vi "EJERCICIO 3.vi"() -> ()   [LabVIEW 2014]
uses:
  Tabcontrolcajero.ctl
  Control 1.ctl
panel:
  out "Tab Control":T1
  out "String 2":string
  out "String":string
  out "Boolean 3":bool
  in  "CARD":bool
  in  "picture":picture
  in  "picture 3":picture
  in  "picture 2":picture
  out "String 3":string
  out "Horizontal Progress Bar":dbl(slide) scale=0.0..100.0
  out "decimal integer string":string
  out "String 4":string
  in  "Contraseña":string
  in  "Aceptar":bool
  out "s? t:f":string
  out "s? t:f 3":string
  out "s? t:f 2":string
  out "String 5":string
  in  "Estado de cuenta":bool
  in  "Compra de tiempo aire":bool
  in  "Retiro de Efectivo":bool
  in  "Pago de Tarjeta de Crédito":bool
  in  "Salir":bool
  out "Crédito Disponible":dbl
  out "Adeudo tarjeta de crédito 2":dbl
  out "String 6":string
  in  "Introduzca la cantidad que desea abonar":dbl
  in  "Aceptar":bool
  in  "Menu":bool
  out "Adeudo de la tarjeta de crédito":dbl
  out "Crédito Disponible":dbl
  out "String 7":string
  in  "$200.00":bool
  in  "$100.00":bool
  in  "$300.00":bool
  in  "$500.00":bool
  in  "Menu":bool
  out "Crédito Disponible":dbl
  out "String 8":string
  in  "Menu":bool
  out "output array 2":string[](array[string])
  out "String 9":string
  in  "Aceptar":bool
  in  "Menu":bool
  in  "Introduzca la cantidad de dinero que desea  retirar":dbl
  out "Crédito Disponible":dbl
  # "0344"
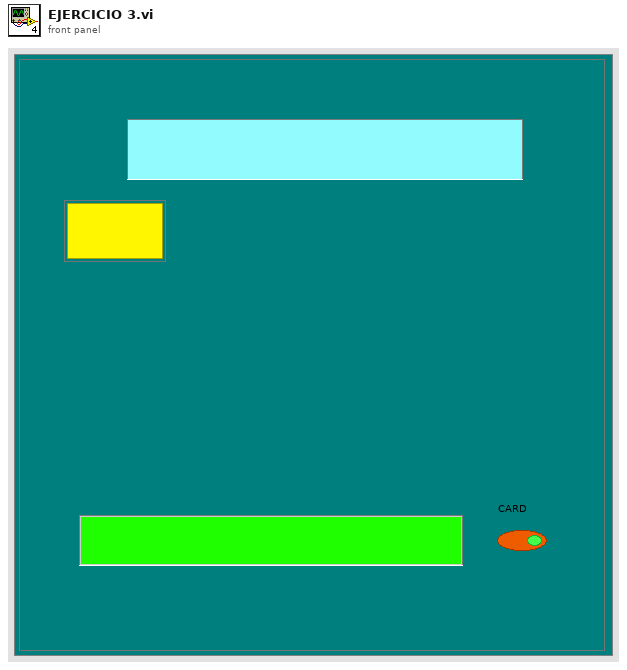
[diagram p1: front panel]
types:
  T1 = typedef "Tabcontrolcajero.ctl" = enum32{"Inicio", "Validacion", "Contraseña", "Menu", "Pago", "Tiempo ", "Cuenta", "Retiro"}
  T2 = typedef "Control 1.ctl" = enum16{"1", "2", "3"}
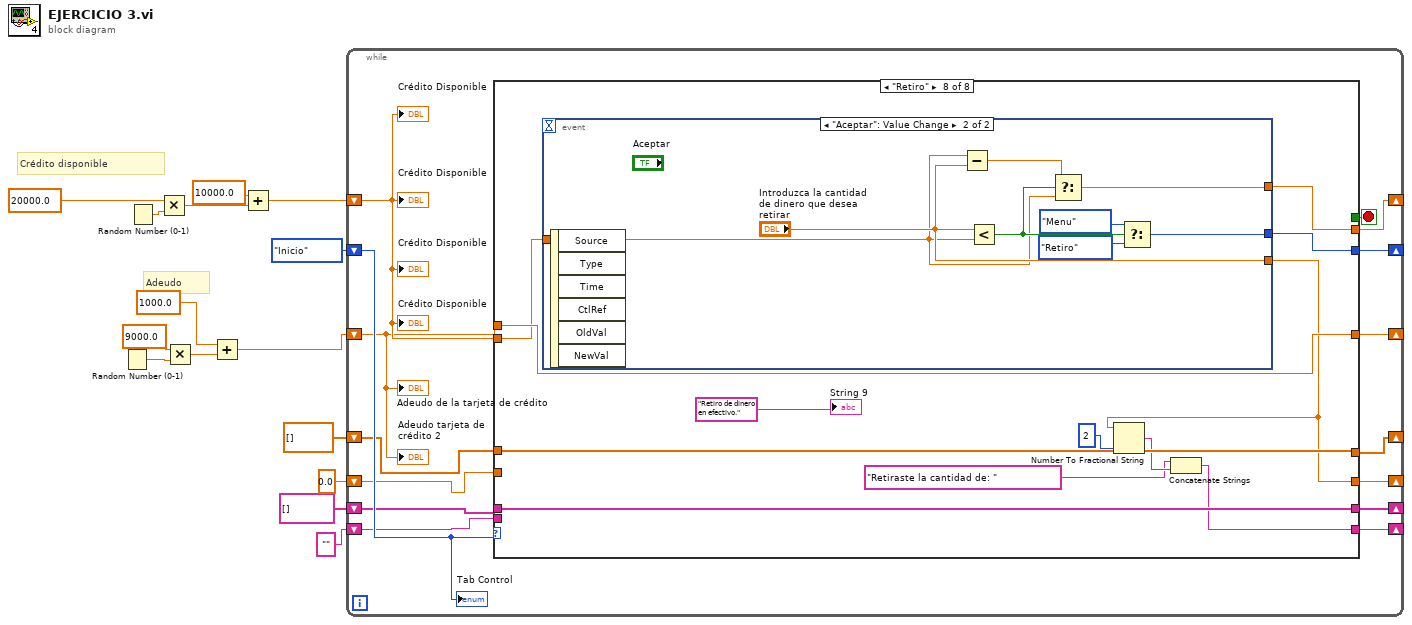
[diagram p0: block diagram]
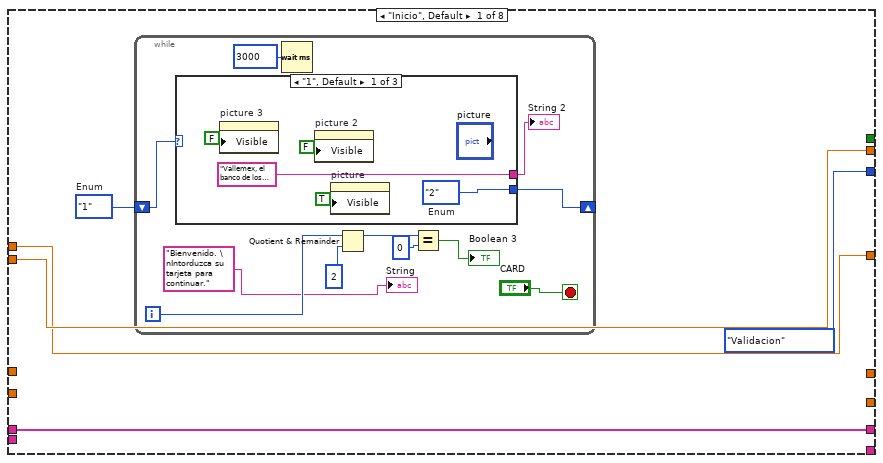
[diagram p2: hidden frame]
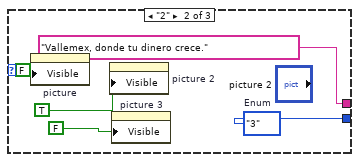
[diagram p3: hidden frame]
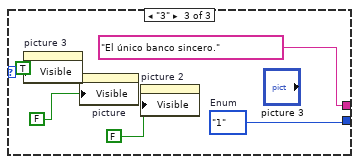
[diagram p4: hidden frame]
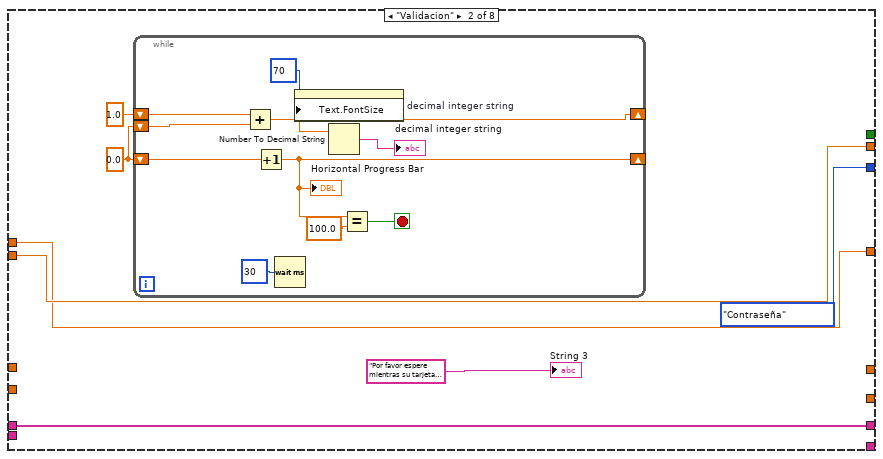
[diagram p5: hidden frame]
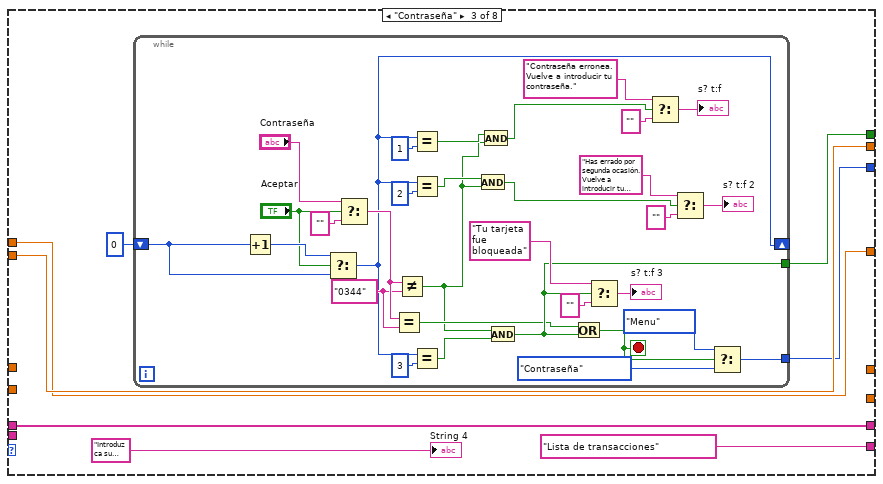
[diagram p6: hidden frame]
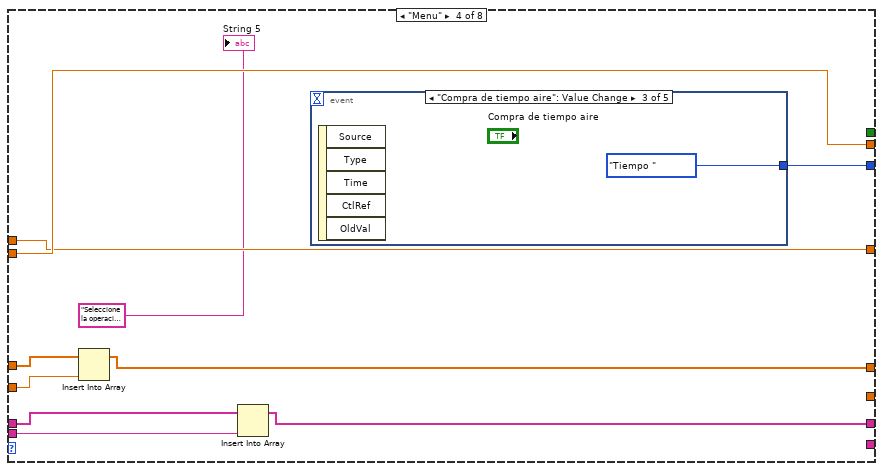
[diagram p7: hidden frame]
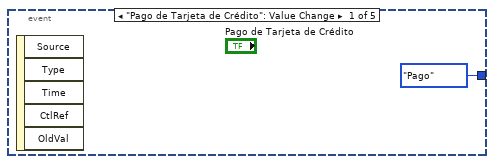
[diagram p8: hidden frame]
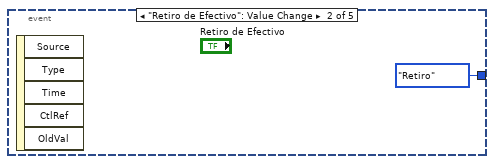
[diagram p9: hidden frame]
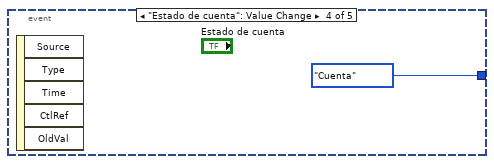
[diagram p10: hidden frame]
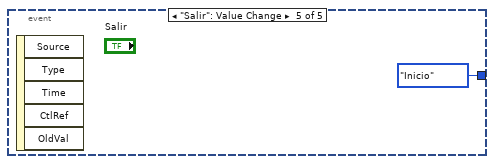
[diagram p11: hidden frame]
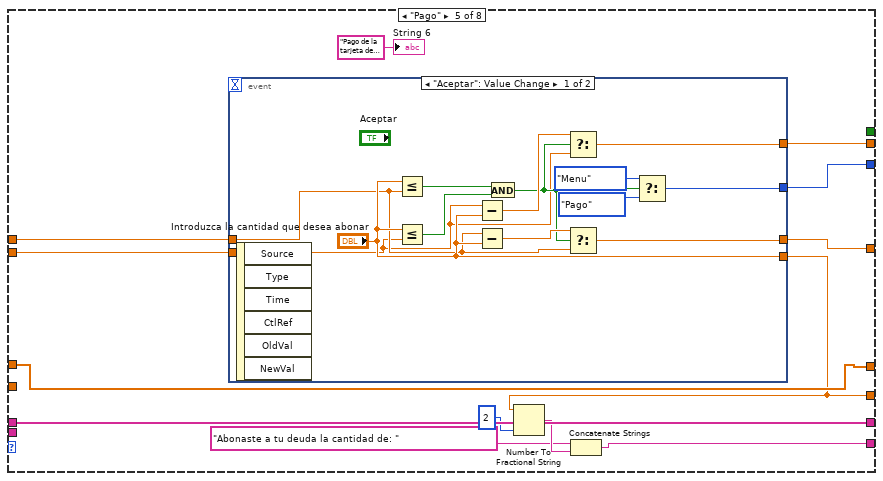
[diagram p12: hidden frame]
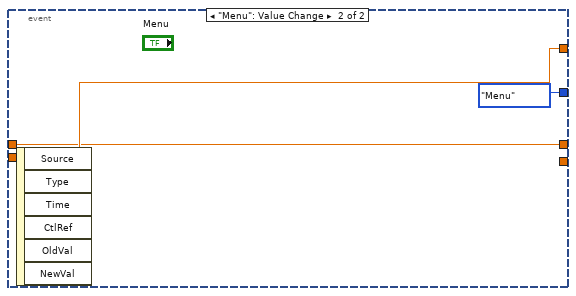
[diagram p13: hidden frame]
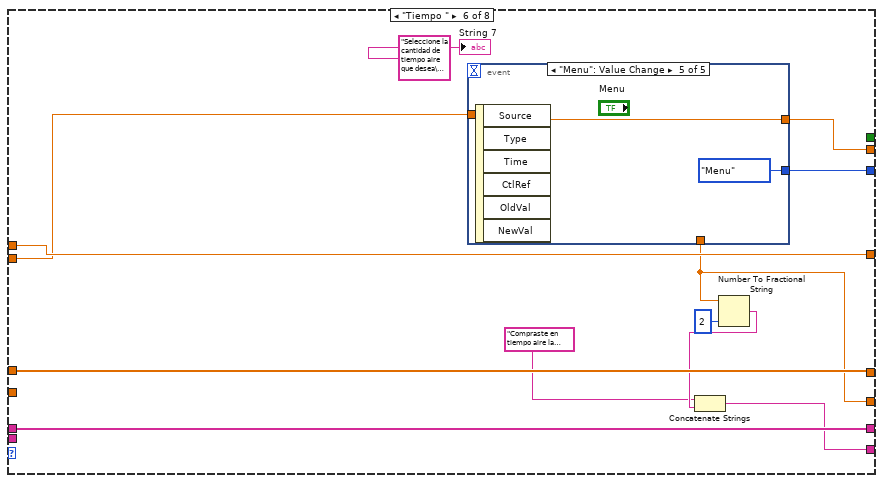
[diagram p14: hidden frame]
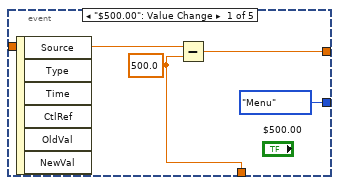
[diagram p15: hidden frame]
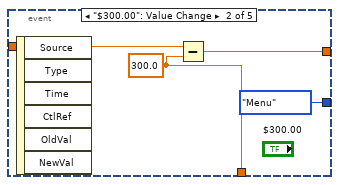
[diagram p16: hidden frame]
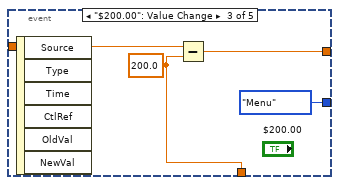
[diagram p17: hidden frame]
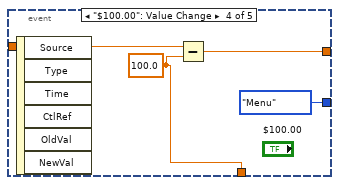
[diagram p18: hidden frame]
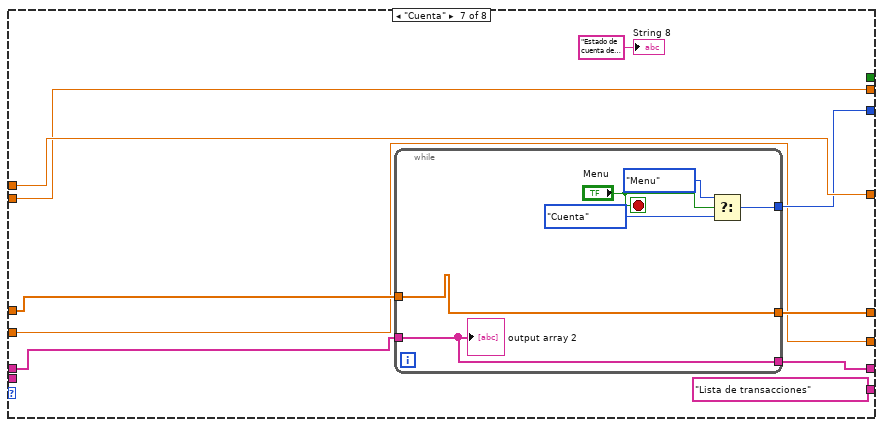
[diagram p19: hidden frame]
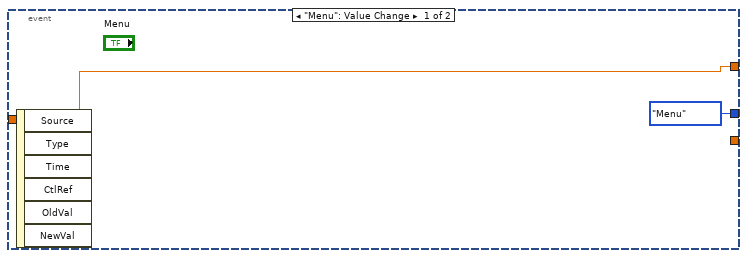
[diagram p20: hidden frame]
diagram:
  # "Adeudo"
  # "Crédito disponible"
  n1 = Random Number (0-1) ("Random Number (10000-30000)")() -> (number: 0 to 1=w10:dbl)
  n2 = Random Number (0-1) ("Random Number (10000-30000)")() -> (number: 0 to 1=w12:dbl)
  n3 = Multiply(x=20000.0, y=w12) -> (x*y=w14:dbl)
  n4 = Multiply(x=9000.0, y=w10) -> (x*y=w8:dbl)
  n5 = Add(x=1000.0, y=w8) -> (x+y=w6:dbl)
  n6 = Add(x=10000.0, y=w14) -> (x+y=w11:dbl)
  n7 = while {
    shift-right: [w30] -> _
    shift-left: w11 -> [w24]
    shift-right: [w29] -> _
    shift-left: w6 -> [w23]
    shift-right: [w28] -> _
    shift-left: Tabcontrolcajero."Inicio" ("Tab Control") -> [w27]
    shift-right: [w25] -> _
    shift-left: dbl[] [] -> [w17]
    shift-right: [w26] -> _
    shift-left: 0.0 ("Introduzca la cantidad a retirar") -> [w19]
    shift-right: [w21] -> _
    shift-left: string[] [] -> [w16]
    shift-right: [w20] -> _
    shift-left: "" -> [w18]
    stop <- w22 stop-if-true
    n8 = case shown="\"Retiro\"" w27 {
      tunnel: [Tabcontrolcajero."Validacion" ("Tab Control") Tabcontrolcajero."Contraseña" ("Tab Control") w82 w128 w146 w172 w201 w220] -> w28
      tunnel: [w35 w66 w86 w127 w142 w171 w200 w217] -> w30
      tunnel: w24 -> [w35 w66 w86 w127 w145 w173 w200 w218]
      tunnel: [w34 w65 w85 w126 w143 w174 w202 w219] -> w29
      tunnel: w23 -> [w34 w65 w85 w126 w144 w174 w202 w219]
      tunnel: [_ _ _ _ w137 w168 w194 w212] -> w26
      tunnel: [_ _ _ w123 w140 w169 w196 w215] -> w25
      tunnel: [_ _ w83 _ _ _ _ _] -> w22
      tunnel: [w32 w63 w81 w120 w141 w170 w195 w216] -> w21
      tunnel: [_ _ "Lista de transacciones" _ w135 w167 "Lista de transacciones" w210] -> w20
      tunnel: w19 -> [_ _ _ w124 _ _ w194 _]
      tunnel: w16 -> [w32 w63 w81 w122 w141 w170 w198 w216]
      tunnel: w17 -> [_ _ _ w125 w140 w169 w199 w215]
      tunnel: w18 -> [_ _ _ w121 _ _ _ _]
      frame "Inicio", Default {
        w31 = Control_1."1"  # Enum
        n9 = while {
          shift-right: [w40] -> _
          shift-left: w31 -> [w39]
          i -> [w38]
          stop <- "CARD" stop-if-true
          n10 = case shown="\"1\", Default" w39 {
            tunnel: [w51 w56 w61] -> w40
            tunnel: ["Vallemex, el banco de los ingenieros." "Vallemex, donde tu dinero crece." "El único banco sincero."] -> w36
            frame "1", Default {
              w51 = Control_1."2"  # Enum
              n11 = property on="picture 3" class="Pict"("Visible"=FALSE) -> ()  [unwired: 2 in, 2 out]
              n12 = property on="picture 2" class="Pict"("Visible"=FALSE) -> ()  [unwired: 2 in, 2 out]
              n13 = property on="picture" class="Pict"("Visible"=TRUE) -> ()  [unwired: 2 in, 2 out]
            }
            frame "2" {
              w56 = Control_1."3"  # Enum
              n14 = property on="picture" class="Pict"("Visible"=FALSE) -> ()  [unwired: 2 in, 2 out]
              n15 = property on="picture 2" class="Pict"("Visible"=TRUE) -> ()  [unwired: 2 in, 2 out]
              n16 = property on="picture 3" class="Pict"("Visible"=FALSE) -> ()  [unwired: 2 in, 2 out]
            }
            frame "3" {
              w61 = Control_1."1"  # Enum
              n17 = property on="picture 3" class="Pict"("Visible"=TRUE) -> ()  [unwired: 2 in, 2 out]
              n18 = property on="picture" class="Pict"("Visible"=FALSE) -> ()  [unwired: 2 in, 2 out]
              n19 = property on="picture 2" class="Pict"("Visible"=FALSE) -> ()  [unwired: 2 in, 2 out]
            }
          }
          "String 2" <- w36
          n20 = Wait (ms)(milliseconds to wait=u32 3000) -> ()  [unwired: 1 out]
          n21 = Quotient & Remainder(x=w38, y=2) -> (x-y*floor(x/y)=w46:i32)  [unwired: 1 out]
          n22 = Equal?(x=w46, y=0) -> (x = y?=→"Boolean 3":bool)
          "String" <- "Bienvenido. \nIntorduzca su tarjeta para continuar."
        }
      }
      frame "Validacion" {
        w68 = 0.0
        n23 = while {
          shift-right: [w73] -> _
          shift-left: w68 -> [w77]
          shift-right: [w71] -> _
          shift-left: 1.0 -> [w76]
          shift-left: w68 -> [w75]
          stop <- w72 stop-if-true
          n24 = Add(x=w76, y=w75) -> (x+y=w71:dbl)
          n25 = Increment(x=w77) -> (x+1=w73:dbl)
          "Horizontal Progress Bar" <- w73
          n26 = Wait (ms)(milliseconds to wait=u32 30) -> ()  [unwired: 1 out]
          n27 = property on="decimal integer string" class="Str"("Text.FontSize"=u32 70 ("Text.Font:Size")) -> ()  [unwired: 2 in, 2 out]
          n28 = Number To Decimal String(number=w71) -> (decimal integer string=→"decimal integer string":string)  [unwired: 1 in]
          n29 = Equal?(x=w73, y=100.0) -> (x = y?=w72:bool)
        }
        "String 3" <- "Por favor espere mientras su tarjeta es validada." ("String 3")
      }
      frame "Contraseña" {
        n30 = while {
          shift-right: [w98] -> _
          shift-left: 0 ("y") -> [w96]
          tunnel: [w104] -> w83
          tunnel: [w100] -> w82
          stop <- w99 stop-if-true
          w113 = "0344"
          n31 = Increment(x=w96) -> (x+1=w97:i32)
          n32 = Select(t=w97, s="Aceptar", f=w96) -> (s? t:f=w98:i32)
          n33 = Select(t="Contraseña", s="Aceptar", f="") -> (s? t:f=w114:string)
          n34 = Equal?(x=w114, y=w113) -> (x = y?=w103:bool)
          n35 = Not Equal?(x=w114, y=w113) -> (x != y?=w89:bool)
          n36 = Equal?(x=w98, y=1) -> (x = y?=w91:bool)
          n37 = Equal?(x=w98, y=2) -> (x = y?=w90:bool)
          n38 = Equal?(x=w98, y=3) -> (x = y?=w111:bool)
          n39 = And(x=w90, y=w89) -> (x .and. y?=w87:bool)
          n40 = And(x=w91, y=w89) -> (x .and. y?=w88:bool)
          n41 = And(x=w89, y=w111) -> (x .and. y?=w104:bool)
          n42 = Or(x=w103, y=w104) -> (x .or. y?=w99:bool)
          n43 = Select(t="Tu tarjeta fue bloqueada", s=w104, f="") -> (s? t:f=→"s? t:f 3":string)
          n44 = Select(t="Contraseña erronea. Vuelve a introducir tu contraseña.", s=w88, f="") -> (s? t:f=→"s? t:f":string)
          n45 = Select(t="Has errado por segunda ocasión. Vuelve a introducir tu contraseña.", s=w87, f="") -> (s? t:f=→"s? t:f 2":string)
          n46 = Select(t=Tabcontrolcajero."Menu" ("Tab Control"), s=w99, f=Tabcontrolcajero."Contraseña" ("Tab Control")) -> (s? t:f=w100:T1)
        }
        "String 4" <- "Introduzca su contraseña de 4 dígitos." ("String 5")
      }
      frame "Menu" {
        n47 = Insert Into Array(array=w125, new element=w124) -> (w123:dbl[])  [unwired: 1 in]
        n48 = Insert Into Array(array=w122, new element=w121) -> (w120:string[])  [unwired: 1 in]
        n49 = event shown="[2] \"Compra de tiempo aire\": Value Change" {
          selector: _ -> [_ _ _ _ _]
          dyn-events: _ -> [_ _ _ _ _]
          timeout: _ -> [_ _ _ _ _]
          tunnel: [Tabcontrolcajero."Pago" ("Tab Control") Tabcontrolcajero."Retiro" ("Tab Control") Tabcontrolcajero."Tiempo " ("Tab Control") Tabcontrolcajero."Cuenta" ("Tab Control") Tabcontrolcajero."Inicio" ("Tab Control")] -> w128
          event "Pago de Tarjeta de Crédito": Value Change {
            n50 = event-data() -> ()  [unwired: 1 in, 5 out]
          }
          event "Retiro de Efectivo": Value Change {
            n51 = event-data() -> ()  [unwired: 1 in, 5 out]
          }
          event "Compra de tiempo aire": Value Change {
            n52 = event-data() -> ()  [unwired: 1 in, 5 out]
          }
          event "Estado de cuenta": Value Change {
            n53 = event-data() -> ()  [unwired: 1 in, 5 out]
          }
          event "Salir": Value Change {
            n54 = event-data() -> ()  [unwired: 1 in, 5 out]
          }
        }
        "String 5" <- "Seleccione la operación que desea realizar." ("String 5")
      }
      frame "Pago" {
        n55 = event shown="[0] \"Aceptar\": Value Change" {
          selector: _ -> [_ _]
          dyn-events: _ -> [_ _]
          timeout: _ -> [_ _]
          tunnel: [w152 Tabcontrolcajero."Menu" ("Tab Control")] -> w146
          tunnel: w145 -> [w147 w161]
          tunnel: w144 -> [w150 w160]
          tunnel: [w156 w160] -> w143
          tunnel: [w148 w161] -> w142
          tunnel: ["Introduzca la cantidad que desea abonar" _] -> w137
          event "Aceptar": Value Change {
            n56 = event-data() -> ()  [unwired: 1 in, 6 out]
            n57 = Less Or Equal?(x="Introduzca la cantidad que desea abonar", y=w150) -> (x <= y?=w158:bool)
            n58 = Less Or Equal?(x="Introduzca la cantidad que desea abonar", y=w147) -> (x <= y?=w159:bool)
            n59 = Subtract(x=w147, y="Introduzca la cantidad que desea abonar") -> (x-y=w151:dbl)
            n60 = Subtract(x=w150, y="Introduzca la cantidad que desea abonar") -> (x-y=w157:dbl)
            n61 = And(x=w158, y=w159) -> (x .and. y?=w149:bool)
            n62 = Select(t=w151, s=w149, f=w147) -> (s? t:f=w148:dbl)
            n63 = Select(t=w157, s=w149, f=w150) -> (s? t:f=w156:dbl)
            n64 = Select(t=Tabcontrolcajero."Menu" ("Tab Control"), s=w149, f=Tabcontrolcajero."Pago" ("Tab Control")) -> (s? t:f=w152:T1)
          }
          event "Menu": Value Change {
            n65 = event-data() -> ()  [unwired: 1 in, 6 out]
          }
        }
        n66 = Number To Fractional String(number=w137, precision (6)=i16 2) -> (F-format string=w139:string)  [unwired: 2 in]
        n67 = Concatenate Strings("Abonaste a tu deuda la cantidad de: ", w139) -> (w135:string)
        "String 6" <- "Pago de la tarjeta de crédito." ("String 6")
      }
      frame "Tiempo " {
        n68 = event shown="[4] \"Menu\": Value Change" {
          selector: _ -> [_ _ _ _ _]
          dyn-events: _ -> [_ _ _ _ _]
          timeout: _ -> [_ _ _ _ _]
          tunnel: w173 -> [w178 w182 w186 w190 w191]
          tunnel: [w177 w181 w185 w189 w191] -> w171
          tunnel: [Tabcontrolcajero."Menu" ("Tab Control") Tabcontrolcajero."Menu" ("Tab Control") Tabcontrolcajero."Menu" ("Tab Control") Tabcontrolcajero."Menu" ("Tab Control") Tabcontrolcajero."Menu" ("Tab Control")] -> w172
          tunnel: [w175 w179 w183 w187 _] -> w168
          event "$500.00": Value Change {
            w175 = 500.0 ("y")
            n69 = event-data() -> ()  [unwired: 1 in, 6 out]
            n70 = Subtract(x=w178, y=w175) -> (x-y=w177:dbl)
          }
          event "$300.00": Value Change {
            w179 = 300.0 ("y")
            n71 = event-data() -> ()  [unwired: 1 in, 6 out]
            n72 = Subtract(x=w182, y=w179) -> (x-y=w181:dbl)
          }
          event "$200.00": Value Change {
            w183 = 200.0 ("y")
            n73 = event-data() -> ()  [unwired: 1 in, 6 out]
            n74 = Subtract(x=w186, y=w183) -> (x-y=w185:dbl)
          }
          event "$100.00": Value Change {
            w187 = 100.0 ("y")
            n75 = event-data() -> ()  [unwired: 1 in, 6 out]
            n76 = Subtract(x=w190, y=w187) -> (x-y=w189:dbl)
          }
          event "Menu": Value Change {
            n77 = event-data() -> ()  [unwired: 1 in, 6 out]
          }
        }
        n78 = Number To Fractional String(number=w168, precision (6)=i16 2) -> (F-format string=w166:string)  [unwired: 2 in]
        n79 = Concatenate Strings("Compraste en tiempo aire la cantidad de: ", w166) -> (w167:string)
        "String 7" <- "Seleccione la cantidad de tiempo aire que desea\nrecargar." ("String 7")
      }
      frame "Cuenta" {
        n80 = while {
          tunnel: [w206] -> w201
          tunnel: w199 -> [w204]
          tunnel: w198 -> [w203]
          tunnel: [w204] -> w196
          tunnel: [w203] -> w195
          stop <- "Menu" stop-if-true
          n81 = Select(t=Tabcontrolcajero."Menu" ("Tab Control"), s="Menu", f=Tabcontrolcajero."Cuenta" ("Tab Control")) -> (s? t:f=w206:T1)
          "output array 2" <- w203
        }
        "String 8" <- "Estado de cuenta del cliente." ("String 8")
      }
      frame "Retiro" {
        n82 = event shown="[1] \"Aceptar\": Value Change" {
          selector: _ -> [_ _]
          dyn-events: _ -> [_ _]
          timeout: _ -> [_ _]
          tunnel: [Tabcontrolcajero."Menu" ("Tab Control") w226] -> w220
          tunnel: w218 -> [w221 w223]
          tunnel: [w221 w225] -> w217
          tunnel: [_ "Introduzca la cantidad de dinero que desea  retirar"] -> w212
          event "Menu": Value Change {
            n83 = event-data() -> ()  [unwired: 1 in, 6 out]
          }
          event "Aceptar": Value Change {
            n84 = event-data() -> ()  [unwired: 1 in, 6 out]
            n85 = Subtract(x=w223, y="Introduzca la cantidad de dinero que desea  retirar") -> (x-y=w227:dbl)
            n86 = Less?(x="Introduzca la cantidad de dinero que desea  retirar", y=w223) -> (x < y?=w230:bool)
            n87 = Select(t=w227, s=w230, f=w223) -> (s? t:f=w225:dbl)
            n88 = Select(t=Tabcontrolcajero."Menu" ("Tab Control"), s=w230, f=Tabcontrolcajero."Retiro" ("Tab Control")) -> (s? t:f=w226:T1)
          }
        }
        n89 = Number To Fractional String(number=w212, precision (6)=i16 2) -> (F-format string=w213:string)  [unwired: 2 in]
        n90 = Concatenate Strings("Retiraste la cantidad de: ", w213) -> (w210:string)
        "String 9" <- "Retiro de dinero en efectivo." ("String 9")
      }
    }
    "Tab Control" <- w27
    "Crédito Disponible" <- w24
    "Crédito Disponible" <- w24
    "Crédito Disponible" <- w24
    "Crédito Disponible" <- w24
    "Adeudo de la tarjeta de crédito" <- w23
    "Adeudo tarjeta de crédito 2" <- w23
  }
